vi "wd_checkAppendError.vi"(8 "error in (no error)":errorcluster) -> (0 "error out":errorcluster, 2 "special error?":bool)   [LabVIEW 2020, in "NI_ExcelFile.lvlib"]
uses:
  <vilib>/express/express shared/NI_ExcelFile/NI_ExcelFile.lvlib
  <vilib>/Utility/error.llb/Error Cluster From Error Code.vi
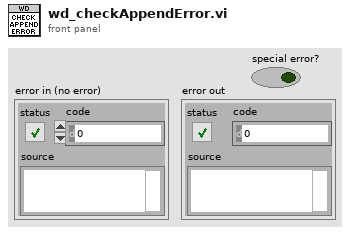
[diagram p1: front panel]
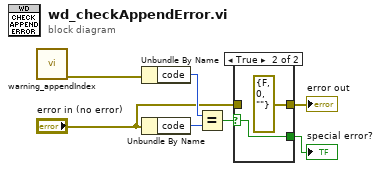
[diagram p0: block diagram]
diagram:
  n1 = call <vilib>:"warning_appendIndex.vi"() -> ("error out"=w5:errorcluster)  [unwired: 11 in]
  n2 = Unbundle By Name(w5) -> ("code"=w6:i32)
  n3 = Unbundle By Name("error in (no error)") -> ("code"=w7:i32)
  n4 = Equal?(x=w6, y=w7) -> (x = y?=w4:bool)
  n5 = case shown="True" w4 {
    selector: w4 -> [w8 w11]
    tunnel: [w8 w11] -> w3
    tunnel: "error in (no error)" -> [w9 _]
    tunnel: [w9 errorcluster {"status"=FALSE, "code"=0, "source"=""} ("error in (no error)")] -> w1
    frame False {
    }
    frame True {
    }
  }
  "special error?" <- w3
  "error out" <- w1
